vi "Popup Message.vi"(1 "error in":errorcluster, 2 "Button Text":string, 3 "Dialogue Message":string) -> (0 "error out":errorcluster)   [LabVIEW 2025]
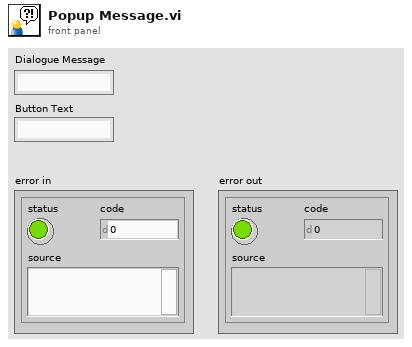
[diagram p1: front panel]
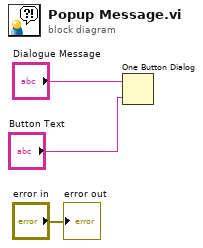
[diagram p0: block diagram]
diagram:
  n1 = One Button Dialog(message="Dialogue Message", button name ("OK")="Button Text") -> ()  [unwired: 1 out]
  "error out" <- "error in"
